vi "SaveImage.vi"(8 "error in (no error)":errorcluster, 10 "ready":bool, 11 "PhotometricsCH250in":refnum<class "Photometrics_CH-250_Cam.lvclass">) -> (0 "error out":errorcluster, 2 "'Save'Command":string, 3 "PhotometricsCH250out":refnum<class "Photometrics_CH-250_Cam.lvclass">)   [LabVIEW 2013, in "Photometrics_CH-250_Cam.lvclass"]
uses:
  Photometrics_CH-250_Cam.lvclass
  Photometrics_CH-250_Cam.lvclass/Photometrics_CH-250_Cam.ctl
  CameraSessionClass/CS250-CameraHardwareClass.lvclass
  shared/CompressAndUpdate(Poly)/CompressAndUpdate(Numeric).vi
  shared/CompressAndUpdate(Poly)/CompressAndUpdate(IMAQ Image).vi
  <vilib>/vision/NI_Vision_Development_Module.lvlib
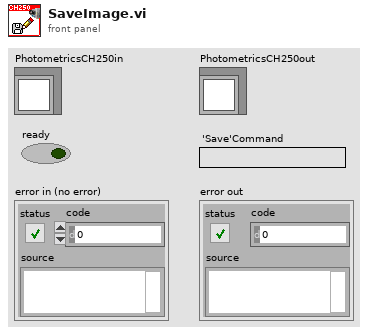
[diagram p1: front panel]
types:
  T1 = typedef "Image Type" = u32
  T2 = typedef "OnOffTypeDef.ctl" = enum16{"off", "on"}
  T3 = typedef "IMAQ Image.ctl" = refnum<image>
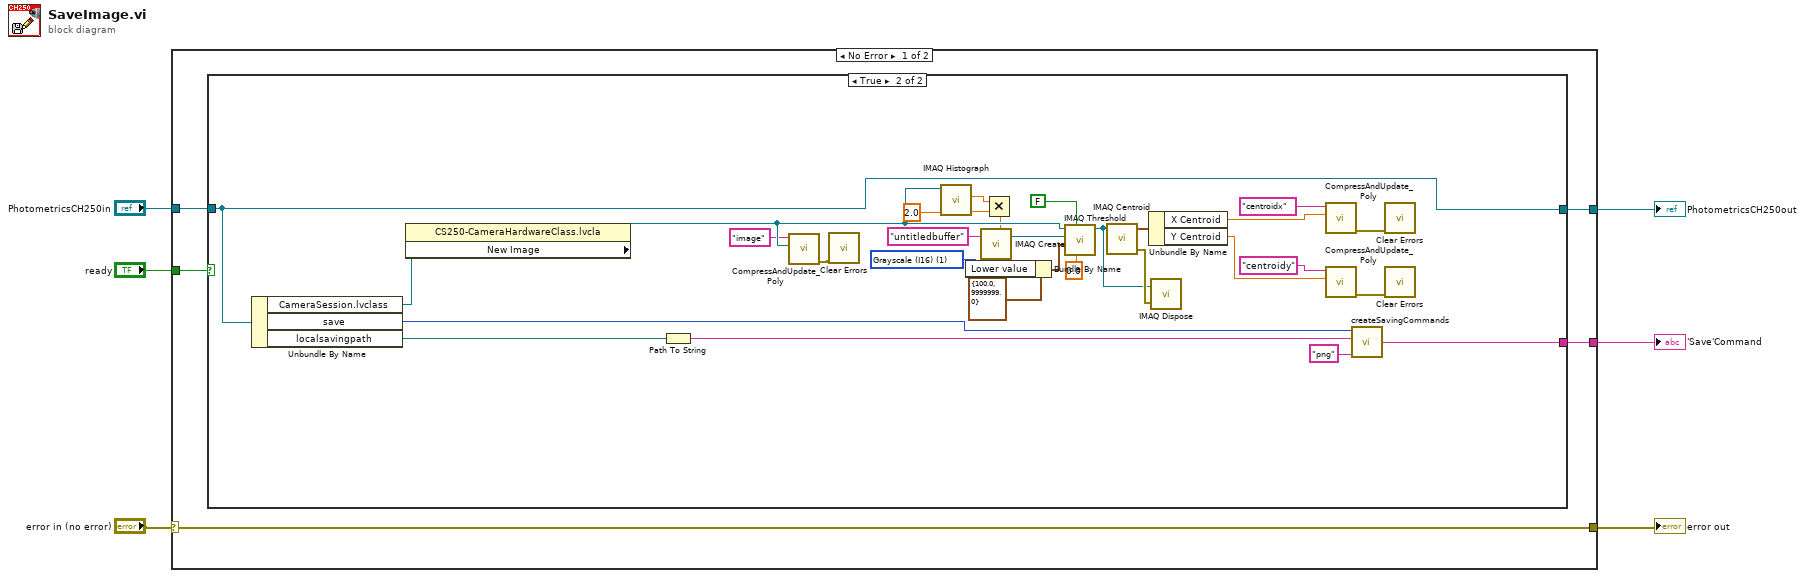
[diagram p0: block diagram]
diagram:
  n1 = case shown="No Error" "error in (no error)" {
    selector: "error in (no error)" -> [w10 w43]
    tunnel: [w11 _] -> w2
    tunnel: "ready" -> [w9 _]
    tunnel: "PhotometricsCH250in" -> [w7 w42]
    tunnel: [w10 w43] -> w6
    tunnel: [w8 w42] -> w1
    frame No Error {
      n2 = case shown="True" w9 {
        tunnel: [_ w40] -> w11
        tunnel: w7 -> [w12 w32]
        tunnel: [w12 w32] -> w8
        frame False {
        }
        frame True {
          w23 = T1 1 items=["Grayscale (U8)", "Grayscale (I16)", "Grayscale (SGL)", "Complex (CSG)", "RGB (U32)", "HSL (U32)", "RGB (U64)", "Grayscale (U16)"] ("Image Type")
          n3 = Unbundle By Name(w32) -> ("CameraSession.lvclass"=w37:refnum<class "CS250-CameraHardwareClass.lvclass">, "save"=w39:T2, "localsavingpath"=w38:path)
          n4 = property class="CS250-CameraHardwareClass.lvcla"(reference=w37) -> ("New Image"=w36:T3)  [unwired: 1 in, 2 out]
          n5 = Path To String(path=w38) -> (string=w41:string)
          n6 = call-poly "CompressAndUpdate_Poly.vi"("IMAQ Image"=w36, "command or variable name"="image") -> ("error out"=w33:errorcluster)  [unwired: 9 in]
          n7 = call <vilib>:"Clear Errors.vi"("error in (no error)"=w33) -> ()  [unwired: 6 in, 1 out]
          n8 = call "IMAQ Histograph"("Image"=w36) -> ("Mean Value"=w17:sgl)  [unwired: 7 in, 3 out]
          n9 = call "IMAQ Create"("Image Name"="untitledbuffer", "Image Type"=w23) -> ("New Image"=w22:T3)  [unwired: 3 in, 1 out]
          n10 = Multiply(x=w17, y=sgl 2.0) -> (x*y=w14:sgl)
          n11 = Bundle By Name(cluster=cluster{"Lower value":sgl, "Upper value":sgl} {"Lower value"=100.0, "Upper value"=9999999.0} ("Range"), "Lower value"=w14) -> (w13:cluster{"Lower value":sgl, "Upper value":sgl})
          n12 = call "IMAQ Threshold"("Replace Value"=sgl 0.0, "Keep/Replace Value (Replace)"=FALSE, "Range"=w13, "Image Dst"=w22, "Image Src"=w36) -> ("Image Dst Out"=w19:T3)  [unwired: 5 in, 1 out]
          n13 = call "IMAQ Centroid"("Image"=w19) -> ("error out"=w20:errorcluster, "Centroid"=w31:cluster{"X Centroid":sgl, "Y Centroid":sgl})  [unwired: 3 in]
          n14 = Unbundle By Name(w31) -> ("X Centroid"=w28:sgl, "Y Centroid"=w27:sgl)
          n15 = call "IMAQ Dispose"("Image"=w19, "error in (no error)"=w20) -> ()  [unwired: 4 in, 1 out]
          n16 = call-poly "CompressAndUpdate_Poly.vi"("Numeric"=w28, "command or variable name"="centroidx") -> ("error out"=w29:errorcluster)  [unwired: 9 in]
          n17 = call-poly "CompressAndUpdate_Poly.vi"("Numeric"=w27, "command or variable name"="centroidy") -> ("error out"=w30:errorcluster)  [unwired: 9 in]
          n18 = call "createSavingCommands.vi"("extension"="png" ("Fileextension"), "Saving Path (local)"=w41, "Save"=w39) -> ("String"=w40:string)  [unwired: 1 in]
          n19 = call <vilib>:"Clear Errors.vi"("error in (no error)"=w29) -> ()  [unwired: 6 in, 1 out]
          n20 = call <vilib>:"Clear Errors.vi"("error in (no error)"=w30) -> ()  [unwired: 6 in, 1 out]
        }
      }
    }
    frame Error {
    }
  }
  "PhotometricsCH250out" <- w1
  "error out" <- w6
  "'Save'Command" <- w2
